vi "get_settings_cluster.vi"(8 "error in (no error)":errorcluster, 11 "ScanModeCN090721ThreeDScan in":refnum<class "ImagingModeDL100901FlexTrajectory.lvclass">) -> (0 "error out":errorcluster, 2 "settings cluster":variant, 3 "ScanModeCN090721ThreeDScan out":refnum<class "ImagingModeDL100901FlexTrajectory.lvclass">)   [LabVIEW 2010, in "ImagingModeDL100901FlexTrajectory.lvclass"]
uses:
  ImagingModeDL100901FlexTrajectory.lvclass
  ImagingModeDL100901FlexTrajectory.lvclass/ImagingModeDL100901FlexTrajectory.ctl
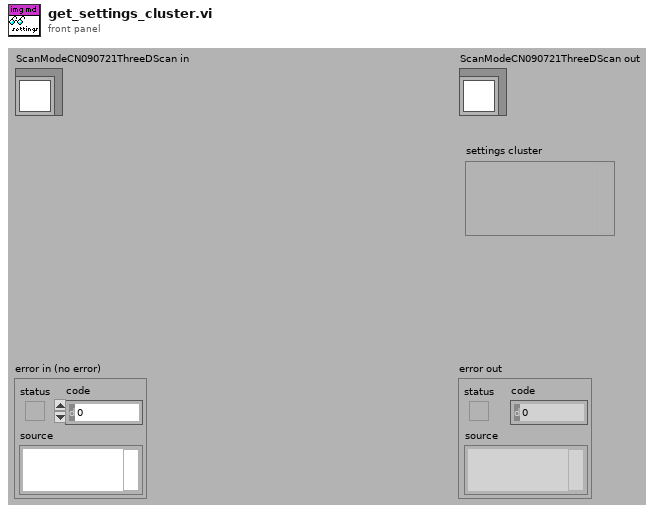
[diagram p1: front panel]
types:
  T1 = typedef "ImagingModeDL100901FlexTrajectory.lvclass/settings_cluster.ctl" = cluster{"ScanRepetitions":i32, "LinesPerFrame":i32, "ScanRate":dbl[unit]}
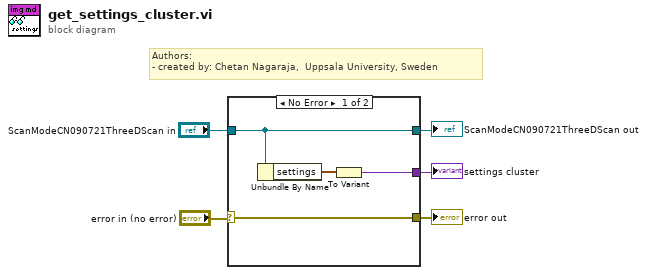
[diagram p0: block diagram]
diagram:
  # "Authors: \n- created by: Chetan Nagaraja,  Uppsala University, Sweden"
  n1 = case shown="No Error" "error in (no error)" {
    selector: "error in (no error)" -> [w7 w11]
    tunnel: [w7 w11] -> w4
    tunnel: "ScanModeCN090721ThreeDScan in" -> [w9 w10]
    tunnel: [w9 w10] -> w2
    tunnel: [w6 _] -> w1
    frame No Error {
      n2 = Unbundle By Name(w9) -> ("settings"=w8:T1)
      n3 = To Variant(anything=w8) -> (Variant=w6:variant)
    }
    frame Error {
    }
  }
  "error out" <- w4
  "ScanModeCN090721ThreeDScan out" <- w2
  "settings cluster" <- w1
